vi "Write Steps Cycle Time.vi"(7 "Send any changes now? (F)":bool, 8 "error in (no error)":errorcluster, 9 "Steps Action":enum16{"Collimation", "Defect detection"}(ring), 10 "Cycle Time":dbl, 11 "Fiber Auto Collimation state data in":refnum<class "Fiber Auto Collimation state data.lvclass">) -> (0 "error out":errorcluster, 3 "Fiber Auto Collimation state data out":refnum<class "Fiber Auto Collimation state data.lvclass">)   [LabVIEW 2018, in "Fiber Auto Collimation state data.lvclass"]
doc: "Serial number of the Device Under Test on the station at the moment."
uses:
  Fiber Auto Collimation state data.lvclass
  Fiber Auto Collimation state data.lvclass/Fiber Auto Collimation state data.ctl
  Tracked state data.ctl
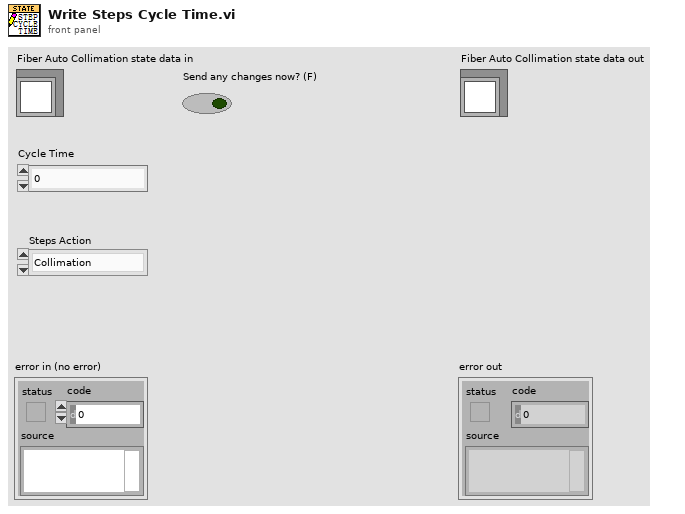
[diagram p1: front panel]
types:
  T1 = typedef "Fiber Auto Collimation state data.lvclass/Tracked state data.ctl" = enum16{"No update", "Permission level", "Username", "Test running", "DUT Serial", "Test status", "MOM Lot", "Loaded test recipe", "Model case running", "Station status", "BV data", "Defect Identify data", "Axis Position data", "Fiber Ass PN", "Operator", "RunTime", "VBAI", "Steps Cycle Time"}
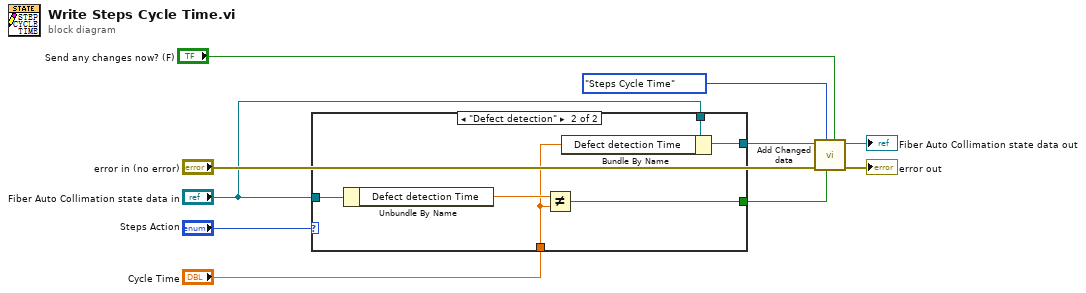
[diagram p0: block diagram]
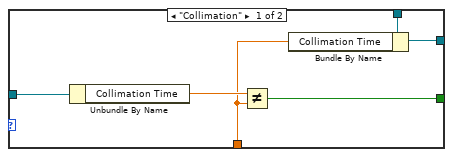
[diagram p2: hidden frame]
diagram:
  n1 = case shown="\"Defect detection\"" "Steps Action" {
    tunnel: "Fiber Auto Collimation state data in" -> [w12 w18]
    tunnel: [w16 w22] -> w8
    tunnel: [w15 w21] -> w5
    tunnel: "Cycle Time" -> [w13 w19]
    tunnel: "Fiber Auto Collimation state data in" -> [w11 w17]
    frame "Collimation" {
      n2 = Unbundle By Name(w12) -> ("Collimation Time"=w14:dbl)
      n3 = Not Equal?(x=w14, y=w13) -> (x != y?=w15:bool)
      n4 = Bundle By Name(cluster=w11, "Collimation Time"=w13) -> (w16:refnum<class "Fiber Auto Collimation state data.lvclass">)
    }
    frame "Defect detection" {
      n5 = Unbundle By Name(w18) -> ("Defect detection Time"=w20:dbl)
      n6 = Not Equal?(x=w20, y=w19) -> (x != y?=w21:bool)
      n7 = Bundle By Name(cluster=w17, "Defect detection Time"=w19) -> (w22:refnum<class "Fiber Auto Collimation state data.lvclass">)
    }
  }
  n8 = call "Add Changed data.vi"("Send any changes now? (F)"="Send any changes now? (F)", "Data changed?"=w5, "Data type"=Tracked_state_data."Steps Cycle Time", "error in (no error)"="error in (no error)", "Fiber Auto Collimation state data in"=w8) -> ("error out"=→"error out":errorcluster, "Fiber Auto Collimation state data out"=→"Fiber Auto Collimation state data out":refnum<class "Fiber Auto Collimation state data.lvclass">)  [unwired: 5 in]
